vi "apply_randomness.vi"(1 "Fraction":dbl, 2 "Input":dbl) -> (0 "Output with noise":dbl)   [LabVIEW 2015]
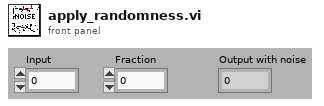
[diagram p1: front panel]
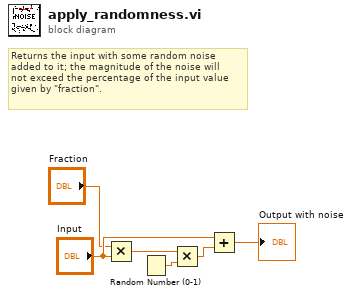
[diagram p0: block diagram]
diagram:
  # "Returns the input with some random noise\nadded to it; the magnitude of the noise will\nnot exceed the percentage of the input value\ngiven by \"fraction\"."
  n1 = Multiply(x="Fraction", y="Input") -> (x*y=w2:dbl)
  n2 = Random Number (0-1)() -> (number: 0 to 1=w1:dbl)
  n3 = Multiply(x=w2, y=w1) -> (x*y=w4:dbl)
  n4 = Add(x="Input", y=w4) -> (x+y=→"Output with noise":dbl)
